vi "ZMC Make Zlib.vi"(8 "error in (no error)":errorcluster caption="错误输入（无错误）", 10 "pfilenameZlb":string, 11 "pfilenameBas":string) -> (0 "error out":errorcluster caption="错误输出", 3 "function return":i32)   [LabVIEW 2015, in "zauxdll.lvlib"]
doc: "int32 __stdcall ZMC_MakeZlib(const char* pfilenameBas, const char* pfilenameZlb);"
uses:
  zauxdll.lvlib
  zmotion.dll
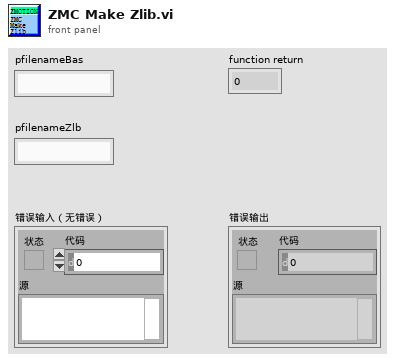
[diagram p1: front panel]
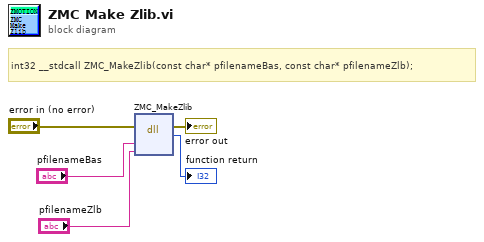
[diagram p0: block diagram]
diagram:
  # "int32 __stdcall ZMC_MakeZlib(const char* pfilenameBas, const char* pfilenameZlb);"
  n1 = dll-call lib="C:/Users/VIC/Desktop/GOGORO_SA/system/LLB/zmotion/zaux/zmotion.*" fn="ZMC_MakeZlib"(error in="error in (no error)", "pfilenameBas"="pfilenameBas", "pfilenameZlb"="pfilenameZlb") -> (error out=→"error out":errorcluster, →"function return":i32)  [unwired: 4 in, 1 out]
